vi "RefreshRequestSummaryinPersonnal.vi"(8 "error in (no error)":errorcluster, 10 "Personnal":string) -> (0 "error out":errorcluster, 2 "Personnal":string)   [LabVIEW 2015]
uses:
  LVClasses/Personnel/Personnel.lvclass/Personnel.ctl
  TypeDef/RequestActionEnum.ctl
  LVClasses/Request/Request.lvclass/Request.ctl
  LVClasses/Request/Read Summary.vi
  LVClasses/Personnel/Read Requests.vi
  LVClasses/Personnel/Write Requests.vi
  LVClasses/Request/Request.lvclass
  LVClasses/Personnel/Personnel.lvclass
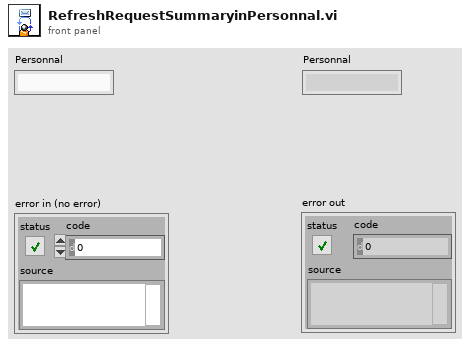
[diagram p1: front panel]
types:
  T1 = typedef "RequestActionEnum.ctl" = enum16{"Init", "ReadRequests", "ReadRequest", "AddRequest", "RemoveRequest", "ToDisk", "Ack", "Complete", "CheckAlarms", "PIntoRoom", "Read Summary", "GetRequestForRoom"}
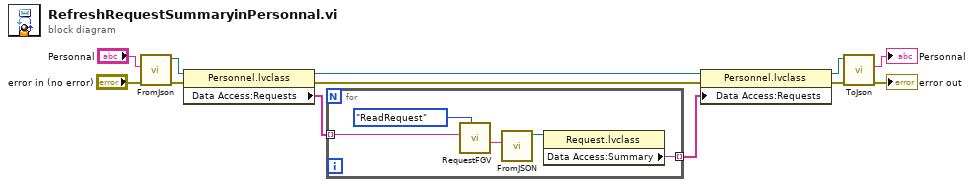
[diagram p0: block diagram]
diagram:
  n1 = call "FromJson.vi"("error in (no error)"="error in (no error)", "PersonnelJson"="Personnal") -> ("error out"=w5:errorcluster, "Personnel out"=w11:refnum<class "Personnel.lvclass">)  [unwired: 8 in]
  n2 = property class="Personnel.lvclass"(reference=w11, error in=w5) -> (reference out=w2:refnum<class "Personnel.lvclass">, error out=w3:errorcluster, "Data Access:Requests"=w4:string[])
  n3 = for {
    tunnel: w4 -> [w17] mode=indexing
    tunnel: [w13] -> w1 mode=indexing
    n4 = call "RequestFGV.vi"("Actions"=RequestActionEnum."ReadRequest", "RUID"=w17) -> ("Data Out"=w14:string)  [unwired: 8 in, 1 out]
    n5 = call "FromJSON.vi"("Request"=w14) -> ("Request out"=w15:refnum<class "Request.lvclass">)  [unwired: 9 in, 1 out]
    n6 = property class="Request.lvclass"(reference=w15) -> ("Data Access:Summary"=w13:string)  [unwired: 1 in, 2 out]
  }
  n7 = property class="Personnel.lvclass"(reference=w2, error in=w3, "Data Access:Requests"=w1) -> (reference out=w10:refnum<class "Personnel.lvclass">, error out=w9:errorcluster)
  n8 = call "ToJson.vi"("error in (no error)"=w9, "Personnel in"=w10) -> ("error out"=→"error out":errorcluster, "PersonnelJson"=→"Personnal":string)  [unwired: 7 in, 1 out]
